vi "Get Primary Destination Path.vi"(8 "error in (no error)":errorcluster, 11 "EXE in":refnum<class "NI_AB_API_EXE.lvclass">) -> (0 "error out":errorcluster, 2 "Primary destination path":path, 3 "EXE out":refnum<class "NI_AB_API_EXE.lvclass">)   [LabVIEW 2020, in "NI_AB_API_EXE.lvclass"]
uses:
  <vilib>/AppBuilder/AB_API/EXE/NI_AB_API_EXE.lvclass
  <vilib>/AppBuilder/AB_API/Application/NI_AB_API_Application.lvclass
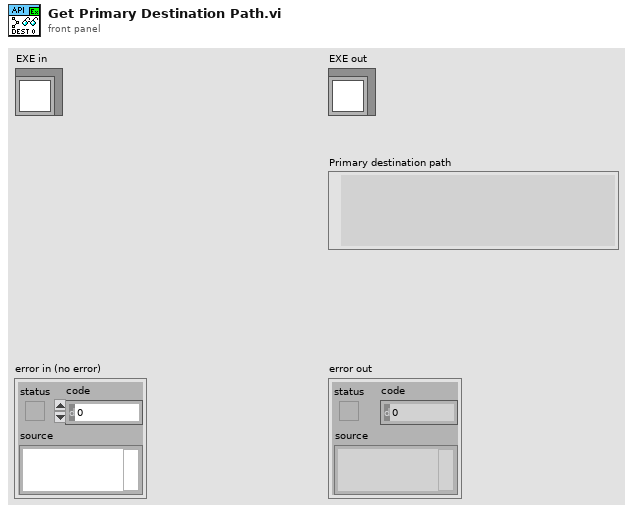
[diagram p1: front panel]
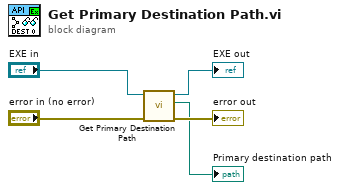
[diagram p0: block diagram]
diagram:
  n1 = call-parent "Get Primary Destination Path.vi"("error in (no error)"="error in (no error)", "NI_AB_API_Build in"="EXE in") -> ("error out"=→"error out":errorcluster, "Primary destination path"=→"Primary destination path":path, "NI_AB_API_Build out"=→"EXE out":refnum<class "NI_AB_API_EXE.lvclass">)  [unwired: 7 in]
